vi "_old_HW_Bundle_Expand_v5.vi"(1 "PB Staging List":T5(array[cluster]), 2 "AO Ramp List":T4(array[cluster]), 3 "Novatech Ramp List":T3(array[cluster]), 4 "DDS Ramp List":T3(array[cluster]), 6 "DDS Devices":T1(array[cluster]), 7 "Number of AO channels":u16, 9 "Number of DO channels":u16, 11 "Number of Novatech channels":u16, 13 "Number of DDS channels":u16) -> (14 "Master Tables":T2)   [LabVIEW 2013]
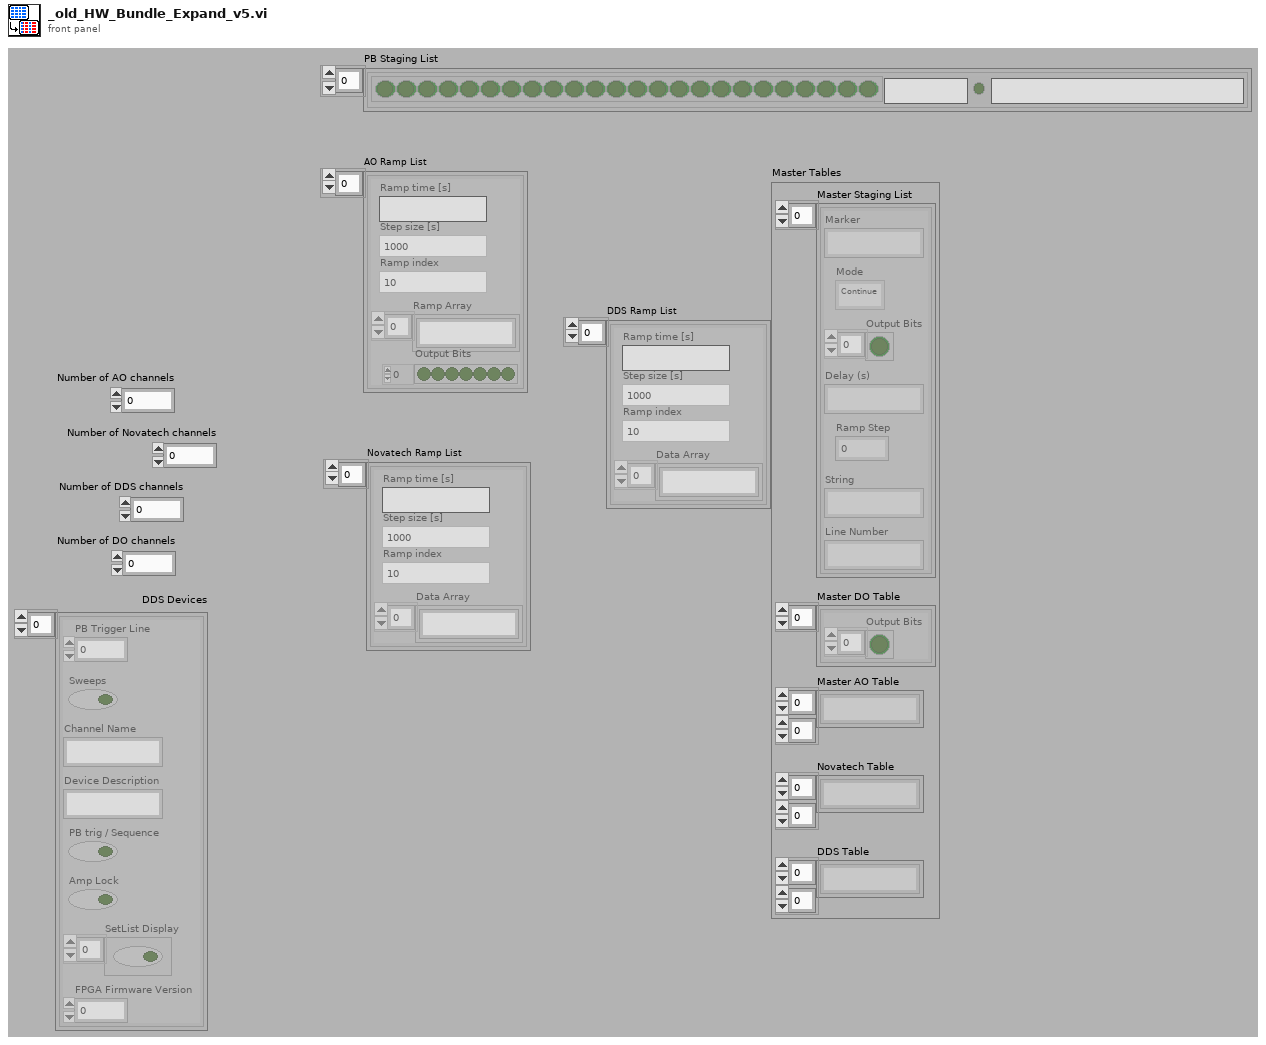
[diagram p1: front panel]
types:
  T1 = cluster{"PB Trigger Line":u16, "Sweeps":bool, "Channel Name":string, "Device Description":string, "PB trig / Sequence":bool, "Amp Lock":bool, "SetList Display":bool[], "FPGA Firmware Version":dbl}[]
  T2 = cluster{"Master Staging List":cluster{"Marker":string, "Mode":enum16{"Continue", "Ramp", "Loop", "EndLoop", "Halt"}, "Output Bits":bool[], "Delay (s)":string, "Ramp Step":dbl, "String":string, "Line Number":string}[], "Master DO Table":cluster{"Output Bits":bool[]}[], "Master AO Table":string[][], "Novatech Table":string[][], "DDS Table":string[][]}
  T3 = cluster{"Ramp index":u32, "Ramp time [s]":string, "Step size [s]":dbl, "Data Array":string[]}[]
  T4 = cluster{"Ramp index":u32, "Ramp time [s]":string, "Step size [s]":dbl, "Ramp Array":string[], "Output Bits":bool[]}[]
  T5 = cluster{"Output Bits":bool[], "Delay (s)":string, "String":string, "Halt?":bool}[]
  T6 = cluster{"Marker":string, "Mode":enum16{"Continue", "Ramp", "Loop", "EndLoop", "Halt"}, "Output Bits":bool[], "Delay (s)":string, "Ramp Step":dbl, "String":string, "Line Number":string}[]
  T7 = cluster{"Marker":string, "Mode":enum16{"Continue", "Ramp", "Loop", "EndLoop", "Halt"}, "Output Bits":bool[], "Delay (s)":string, "Ramp Step":dbl, "String":string, "Line Number":string}
  T8 = enum16{"Continue", "Ramp", "Loop", "EndLoop", "Halt"}
  T9 = cluster{"Ramp index":u32, "Ramp time [s]":string, "Step size [s]":dbl, "Data Array":string[]}
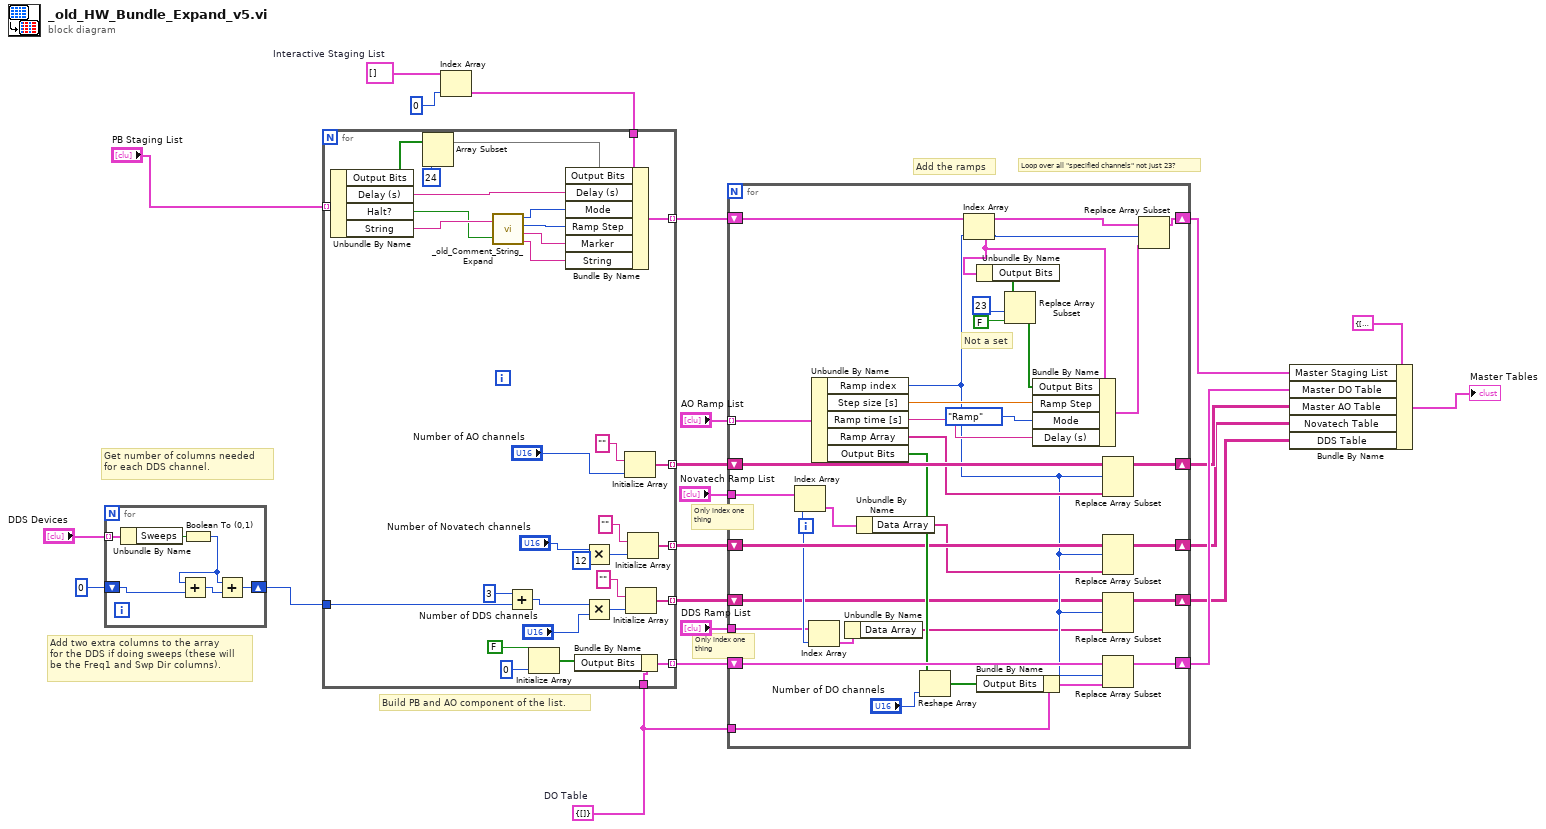
[diagram p0: block diagram]
diagram:
  w2 = cluster{"Output Bits":bool[]} {"Output Bits"=[]}  # DO Table
  w4 = T6 []  # Interactive Staging List
  # "Only index one\nthing"
  # "Get number of columns needed\nfor each DDS channel."
  # "Add two extra columns to the array\nfor the DDS if doing sweeps (these will\nbe the Freq1 and Swp Dir columns)."
  # "Loop over all \"specified channels\" not just 23?"
  # "Only index one\nthing"
  # "Add the ramps"
  # "Build PB and AO component of the list."
  n1 = for {
    tunnel: "DDS Devices" -> [w29] mode=indexing
    shift-right: [w27] -> w13
    shift-left: i16 0 -> [w26]
    n2 = Unbundle By Name(w29) -> ("Sweeps"=w28:bool)
    n3 = Boolean To (0,1)(Boolean=w28) -> (0, 1=w24:i16)
    n4 = Add(x=w24, y=w26) -> (x+y=w25:i16)
    n5 = Add(x=w24, y=w25) -> (x+y=w27:i16)
  }
  n6 = Index Array(array=w4, index=0) -> (element=w18:T7)
  n7 = for {
    tunnel: [w62] -> w21 mode=indexing
    tunnel: "PB Staging List" -> [w59] mode=indexing
    tunnel: w18 -> [w60]
    tunnel: [w49] -> w20 mode=indexing
    tunnel: w2 -> [w45]
    tunnel: [w46] -> w17 mode=indexing
    tunnel: [w42] -> w15 mode=indexing
    tunnel: w13 -> [w36]
    tunnel: [w37] -> w12 mode=indexing
    n8 = Unbundle By Name(w59) -> ("Output Bits"=w58:bool[], "Delay (s)"=w61:string, "Halt?"=w51:bool, "String"=w55:string)
    n9 = Array Subset(array=w58, length=24) -> (w57:bool[])  [unwired: 1 in]
    n10 = call "_old_Comment_String_Expand.vi"("Intial Comment String"=w55, "Halt"=w51) -> ("Option"=w52:T8, "Loops"=w33:u32, "Marker String"=w53:string, "Final Comment String"=w54:string)
    n11 = Add(x=i16 3, y=w36) -> (x+y=w34:i16)
    n12 = Initialize Array(FALSE, 0) -> (w47:bool[])
    n13 = Bundle By Name(cluster=w60, "Output Bits"=w57, "Delay (s)"=w61, "Mode"=w52, "Ramp Step"=w33, "Marker"=w53, "String"=w54) -> (w62:T7)
    n14 = Bundle By Name(cluster=w45, "Output Bits"=w47) -> (w46:cluster{"Output Bits":bool[]})
    n15 = Multiply(x="Number of Novatech channels", y=12) -> (x*y=w40:i32)
    n16 = Multiply(x=w34, y="Number of DDS channels") -> (x*y=w38:u16)
    n17 = Initialize Array("", "Number of AO channels") -> (w49:string[])
    n18 = Initialize Array("", w38) -> (w37:string[])
    n19 = Initialize Array("", w40) -> (w42:string[])
  }
  n20 = for {
    shift-right: [w93] -> w9
    shift-left: w21 -> [w94]
    tunnel: "AO Ramp List" -> [w96] mode=indexing
    shift-right: [w85] -> w7
    shift-left: w20 -> [w86]
    shift-right: [w82] -> w8
    shift-left: w17 -> [w83]
    tunnel: w2 -> [w80]
    tunnel: "Novatech Ramp List" -> [w76]
    shift-right: [w74] -> w6
    shift-left: w15 -> [w73]
    shift-right: [w65] -> w5
    shift-left: w12 -> [w66]
    tunnel: "DDS Ramp List" -> [w69]
    i -> [w71]
    # "Not a set"
    n21 = Index Array(array=w76, index=w71) -> (element=w75:T9)
    n22 = Index Array(array=w69, index=w71) -> (element=w70:T9)
    n23 = Unbundle By Name(w96) -> ("Ramp index"=w68:u32, "Step size [s]"=w92:dbl, "Ramp time [s]"=w95:string, "Ramp Array"=w84:string[], "Output Bits"=w78:bool[])
    n24 = Unbundle By Name(w70) -> ("Data Array"=w67:string[])
    n25 = Unbundle By Name(w75) -> ("Data Array"=w72:string[])
    n26 = Reshape Array(w78, "Number of DO channels") -> (w79:bool[])
    n27 = Index Array(array=w94, index=w68) -> (element=w91:T7)
    n28 = Unbundle By Name(w91) -> ("Output Bits"=w89:bool[])
    n29 = Bundle By Name(cluster=w80, "Output Bits"=w79) -> (w81:cluster{"Output Bits":bool[]})
    n30 = Replace Array Subset(array=w89, new element=FALSE, index=23) -> (w90:bool[])
    n31 = Bundle By Name(cluster=w91, "Output Bits"=w90, "Ramp Step"=w92, "Mode"=T8."Ramp" ("Option 2"), "Delay (s)"=w95) -> (w63:T7)
    n32 = Replace Array Subset(array=w86, new element=w84, index (row)=w68) -> (w85:string[][])  [unwired: 1 in]
    n33 = Replace Array Subset(array=w73, new element=w72, index (row)=w68) -> (w74:string[][])  [unwired: 1 in]
    n34 = Replace Array Subset(array=w66, new element=w67, index (row)=w68) -> (w65:string[][])  [unwired: 1 in]
    n35 = Replace Array Subset(array=w83, new element=w81, index=w68) -> (w82:cluster{"Output Bits":bool[]}[])
    n36 = Replace Array Subset(array=w94, new element=w63, index=w68) -> (w93:T6)
  }
  n37 = Bundle By Name(cluster=T2 {"Master Staging List"=[], "Master DO Table"=[], "Master AO Table"=[], "Novatech Table"=[], "DDS Table"=[]} ("Master Table Tables"), "Master Staging List"=w9, "Master DO Table"=w8, "Master AO Table"=w7, "Novatech Table"=w6, "DDS Table"=w5) -> (→"Master Tables":T2)
